vi "Write Characters To File (with error out).vi"(2 "convert eol? (no:F)":bool, 6 "advisory dialog? (display:T)":bool=TRUE, 7 "pattern":string, 8 "error in (no error)":errorcluster, 9 "append to file? (new file:F)":bool, 10 "character string":string, 11 "file path (dialog if empty)":path) -> (0 "error out":errorcluster, 3 "new file path (Not A Path if cancelled)":path)   [LabVIEW 2012]
doc: "Writes a character string to a new byte stream file or appends the string to an existing file. The VI opens or creates the file beforehand and closes it afterwards.\n\nfile path is the path name of the file. If file path is empty (default value) or is Not A Path, the VI displays a File dialog box from which you can select a file. Error 43 occurs if the user cancels the dialog. \n\ncharacter string is the data the VI writes to the file.\n\nappend to file? Set to TRUE if you want to append the data to a existing file; you can also set it TRUE to write to a new file. Set to FALSE (default value) if you want to write the data to a new file or to replace an existing file.\n\nnew file path is the path of the file to which the VI wrote data. You can use this output to determine the path of a file that you open using dialog. new file path returns Not A Path if the user selects Cancel from the dialog box."
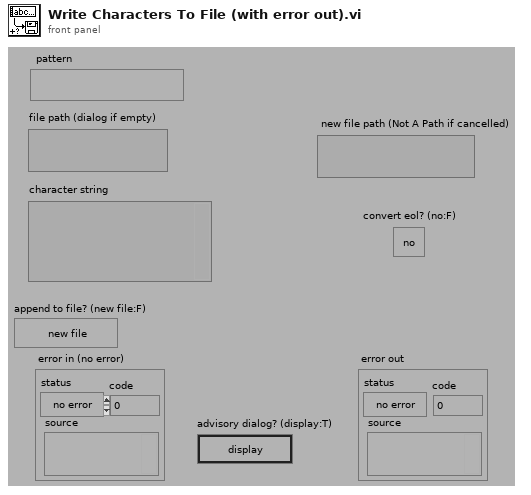
[diagram p1: front panel]
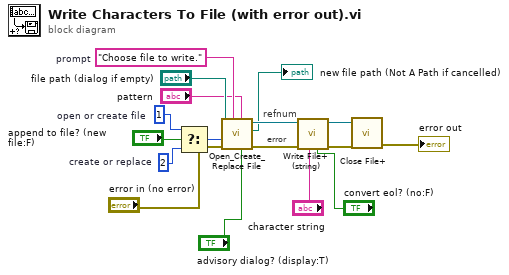
[diagram p0: block diagram]
diagram:
  w8 = i16 2  # create or replace
  w13 = "Choose file to write."  # prompt
  w11 = i16 1  # open or create file
  # "error"
  # "refnum"
  n1 = Select(t=w11, s="append to file? (new file:F)", f=w8) -> (s? t:f=w12:i16)
  n2 = call <vilib>:"Open_Create_Replace File.vi"("advisory dialog? (display:T)"="advisory dialog? (display:T)", "pattern"="pattern", "prompt"=w13, "error in (no error)"="error in (no error)", "function (open:0)"=w12, "file path"="file path (dialog if empty)") -> ("error out"=w16:errorcluster, "new file path"=→"new file path (Not A Path if cancelled)":path, "refnum"=w7:refnum<file>)  [unwired: 2 in, 1 out]
  n3 = call <vilib>:"Write File+ (string).vi"("convert eol? (no:F)"="convert eol? (no:F)", "string"="character string", "error in (no error)"=w16, "refnum"=w7) -> ("error out"=w15:errorcluster, "dup refnum"=w14:refnum<file>)  [unwired: 2 in, 2 out]
  n4 = call <vilib>:"Close File+.vi"("error in (no error)"=w15, "refnum"=w14) -> ("error out"=→"error out":errorcluster)  [unwired: 5 out]
